vi "Read SPL Comment.vi"(8 "error in (no error)":errorcluster, 11 "Filename":path=path "E:/LabVIEW/Data/Test Data/Subj-Austin_Trial-1_Condition-None.lvm") -> (0 "error out":errorcluster, 1 "Signals":string[](array[string]), 2 "Upper SPL":dbl, 3 "Filename Out":path, 5 "Comment":string)   [LabVIEW 2020]
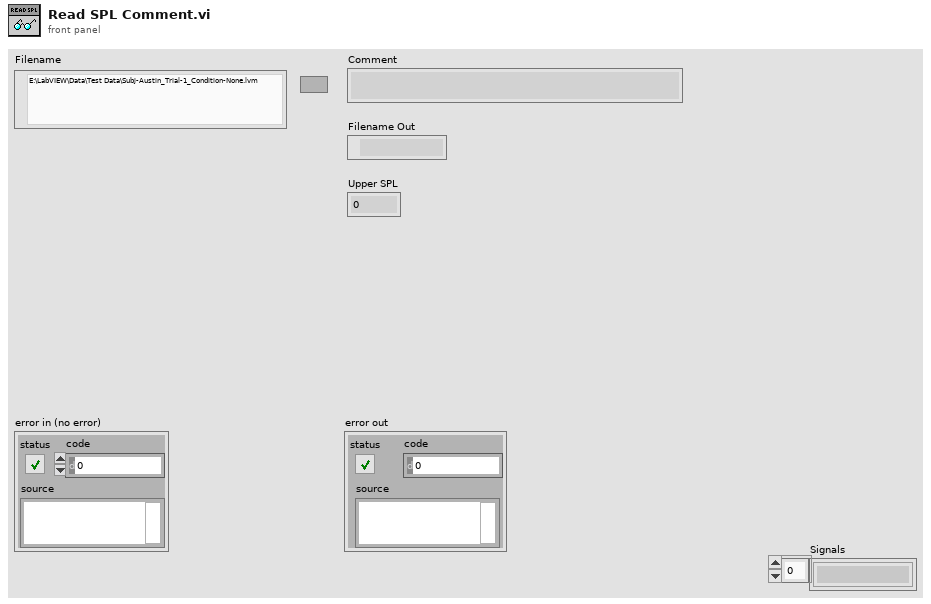
[diagram p1: front panel]
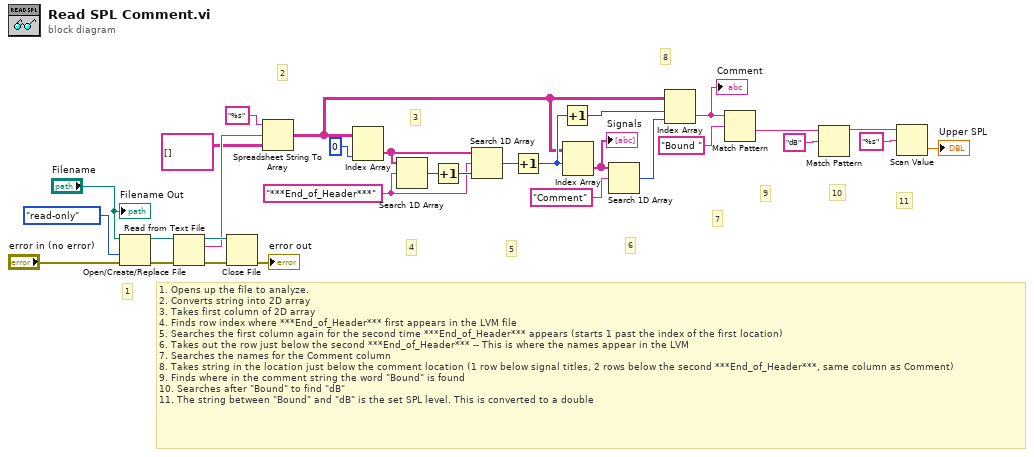
[diagram p0: block diagram]
diagram:
  w10 = "***End_of_Header***" ("element")
  # "11"
  # "10"
  # "9"
  # "8"
  # "7"
  # "6"
  # "5"
  # "4"
  # "3"
  # "2"
  # "1"
  # "1. Opens up the file to analyze.\n2. Converts string into 2D array\n3. Takes first column of 2D array\n4. Finds row index where ***End_of_Header*** first appears in the LVM file\n5. Searches the first column again for the second time ***End_of_Header*** appears (starts 1 past the index of the first location)\n6. Takes out the row just below the second ***End_of_Header*** -- This is where the names appear in the LVM\n7. Searches the names for the Comment column\n8. Takes string in the location just below the comment location (1 row below signal titles, 2 rows below the second ***End_of_Header***, same column as Comment)\n9. Finds where in the comment string the word \"Bound\" is found\n10. Searches after \"Bound\" to find \"dB\"\n11. The string between \"Bound\" and \"dB\" is the set SPL level. This is converted to a double"
  n1 = Open/Create/Replace File(file path (use dialog)="Filename", error in="error in (no error)", access (0:read/write)=enum16{"read/write", "read-only", "write-only"}."read-only") -> (refnum out=w24:refnum<file>, error out=w23:errorcluster)  [unwired: 3 in, 1 out]
  n2 = Read from Text File(file (use dialog)=w24, error in=w23) -> (refnum out=w19:refnum<file>, text=w17:string, error out=w22:errorcluster)  [unwired: 2 in, 1 out]
  n3 = Close File(refnum=w19, error in=w22) -> (error out=→"error out":errorcluster)  [unwired: 1 out]
  n4 = Spreadsheet String To Array(format string="%s", spreadsheet string=w17, array type (2D Dbl)=string[][] []) -> (array=w3:string[][])  [unwired: 1 in]
  n5 = Index Array(array=w3, index (col)=0 ("disabled index (col)")) -> (element=w11:string[])  [unwired: 1 in]
  n6 = Search 1D Array(1D array=w11, element=w10) -> (index of element=w13:i32)  [unwired: 1 in]
  n7 = Increment(x=w13) -> (x+1=w12:i32)
  n8 = Search 1D Array(1D array=w11, element=w10, start index (0)=w12) -> (index of element=w9:i32)
  n9 = Increment(x=w9) -> (x+1=w5:i32)
  n10 = Increment(x=w5) -> (x+1=w4:i32)
  n11 = Index Array(array=w3, index (row)=w5) -> (element=w8:string[])  [unwired: 1 in]
  "Signals" <- w8
  n12 = Search 1D Array(1D array=w8, element="Comment") -> (index of element=w6:i32)  [unwired: 1 in]
  n13 = Index Array(array=w3, index (row)=w4, index (col)=w6) -> (element=w2:string)
  "Comment" <- w2
  n14 = Match Pattern(string=w2, regular expression="Bound ") -> (after substring=w26:string)  [unwired: 1 in, 3 out]
  n15 = Match Pattern(string=w26, regular expression="dB") -> (before substring=w28:string)  [unwired: 1 in, 3 out]
  n16 = Scan Value(string=w28, format string="%s") -> (value=→"Upper SPL":dbl)  [unwired: 1 in, 1 out]
  "Filename Out" <- "Filename"
